vi "SamZ_Format.vi"(11 "Files in":T2[](array[typedef])) -> (3 "Files out":T2[](array[typedef]))   [LabVIEW 2022 SP3]
uses:
  Curtin1_Label.ctl
panel:
  in  "Delays":T1={"time bt taps"=0.5, "time bt positions"=1.0, "time bt sets"=2.0}
  out "Array":path[](array[path])
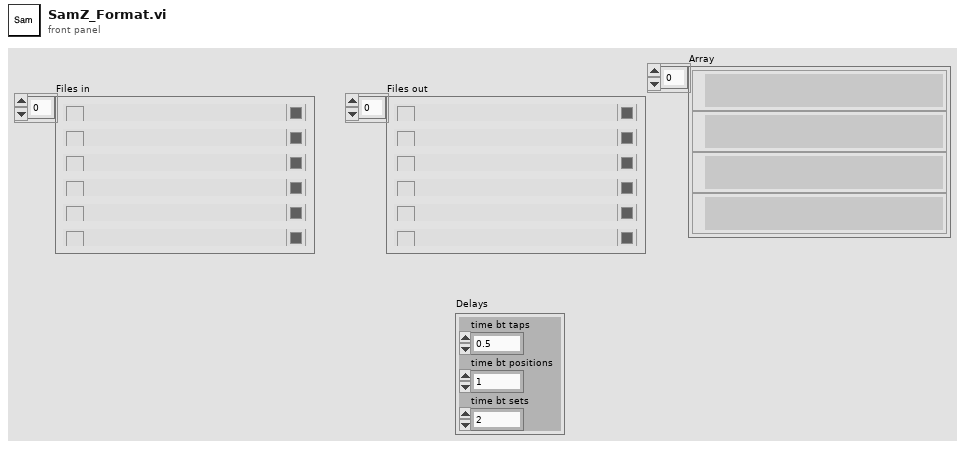
[diagram p1: front panel]
types:
  T1 = cluster{"time bt taps":dbl, "time bt positions":dbl, "time bt sets":dbl}
  T2 = typedef "Curtin1_Label.ctl" = cluster{"Show?":bool, "Name":string, "Color":u32, "Path":path, "Show Notes":bool}
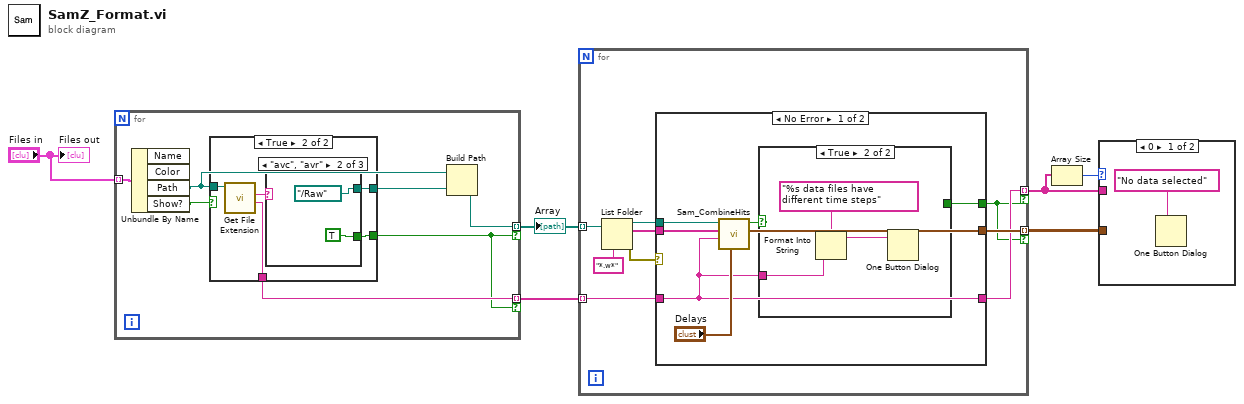
[diagram p0: block diagram]
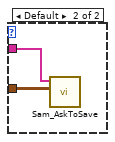
[diagram p2: hidden frame]
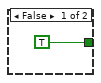
[diagram p3: hidden frame]
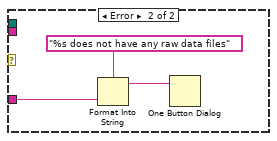
[diagram p4: hidden frame]
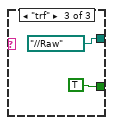
[diagram p7: hidden frame]
diagram:
  n1 = for {
    tunnel: "Files in" -> [w13] mode=indexing
    tunnel: [w10] -> w5 mode=indexing if=w8
    tunnel: [w9] -> w4 mode=indexing if=w8
    n2 = Unbundle By Name(w13) -> ("Path"=w11:path, "Show?"=w12:bool)  [unwired: 2 out]
    n3 = case shown="True" w12 {
      tunnel: w11 -> [_ w17]
      tunnel: [_ w16] -> w8
      tunnel: [_ w15] -> w9
      tunnel: [_ w14] -> w7
      frame False {
      }
      frame True {
        n4 = call <vilib>:"Get File Extension.vi"("file"=w17) -> ("filename without extension"=w15:string, "lowercase file extension"=w18:string)  [unwired: 6 in, 3 out]
        n5 = case shown="\"avc\", \"avr\"" w18 {
          tunnel: [_ TRUE TRUE] -> w16
          tunnel: [_ path "../Raw" ("name or relative path") path "../../Raw" ("name or relative path")] -> w14
          frame Default {
          }
          frame "avc", "avr" {
          }
          frame "trf" {
          }
        }
      }
    }
    n6 = Build Path(base path=w11, name or relative path=w7) -> (appended path=w10:path)
  }
  "Array" <- w5
  n7 = for {
    tunnel: w5 -> [w31] mode=indexing
    tunnel: w4 -> [w27] mode=indexing
    tunnel: [w25] -> w3 mode=indexing if=w23
    tunnel: [w24] -> w1 mode=indexing if=w23
    n8 = List Folder(path=w31, pattern="*.w*") -> (path out=w29:path, filenames=w28:string[], error out=w26:errorcluster)  [unwired: 2 in, 1 out]
    n9 = case shown="No Error" w26 {
      tunnel: w29 -> [w38 _]
      tunnel: w28 -> [w37 _]
      tunnel: w27 -> [w33 w44]
      tunnel: [w32 _] -> w25
      tunnel: [w33 _] -> w24
      tunnel: [w35 _] -> w23
      frame No Error {
        n10 = call "Sam_CombineHits.vi"("Delays"="Delays", "run name"=w33, "raw files"=w37, "raw path"=w38) -> ("Data"=w32:waveform(dbl)[], "dt bad?"=w36:bool)  [unwired: 6 in]
        n11 = case shown="True" w36 {
          tunnel: w33 -> [_ w40]
          tunnel: [TRUE _] -> w35
          frame False {
          }
          frame True {
            n12 = Format Into String(format string="%s data files have different time steps", w40) -> (resulting string=w41:string)  [unwired: 2 in, 1 out]
            n13 = One Button Dialog(message=w41) -> ()  [unwired: 1 in, 1 out]
          }
        }
      }
      frame Error {
        n14 = Format Into String(format string="%s does not have any raw data files", w44) -> (resulting string=w43:string)  [unwired: 2 in, 1 out]
        n15 = One Button Dialog(message=w43) -> ()  [unwired: 1 in, 1 out]
      }
    }
  }
  n16 = Array Size(array=w1) -> (size(s)=w2:i32)
  n17 = case shown="0" w2 {
    tunnel: w1 -> [_ w48]
    tunnel: w3 -> [_ w47]
    frame 0 {
      n18 = One Button Dialog(message="No data selected") -> ()  [unwired: 1 in, 1 out]
    }
    frame Default {
      n19 = call "Sam_AskToSave.vi"("Data"=w47, "Names"=w48) -> ()  [unwired: 10 in]
    }
  }
  "Files out" <- "Files in"
